vi "Update Dictionary.vi"(8 "error in (no error)":errorcluster, 9 "Variant":variant, 10 "Key":string, 11 "SMO.Dictionary in":refnum<class "SMO.Dictionary.lvclass">) -> (0 "error out":errorcluster, 3 "SMO.Dictionary out":refnum<class "SMO.Dictionary.lvclass">)   [LabVIEW 2013, in "SMO.Dictionary.lvlib" / "SMO.Dictionary.lvclass"]
uses:
  SMO.Dictionary.lvclass
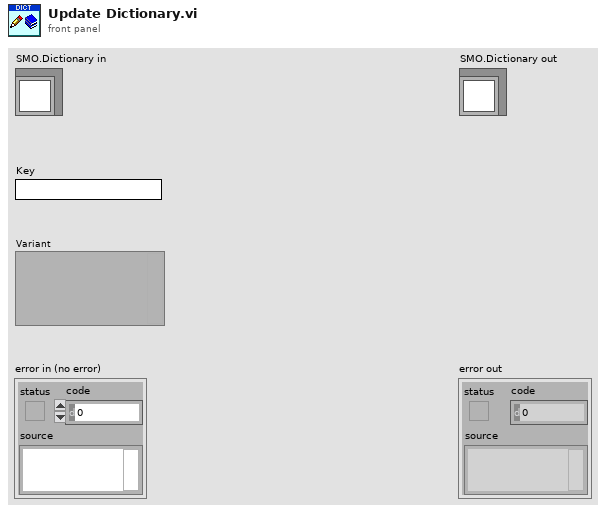
[diagram p1: front panel]
types:
  T1 = typedef "SMO.Dictionary.lvlib/SMO.Dictionary.lvclass/PublicEvents--Cluster.ctl" = cluster{"Cleared":refnum<user-event>, "Deleted":refnum<user-event>, "Updated":refnum<user-event>}
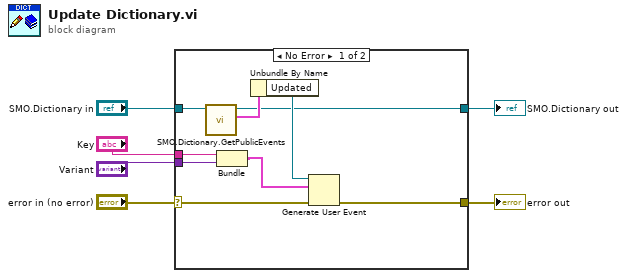
[diagram p0: block diagram]
diagram:
  n1 = case shown="No Error" "error in (no error)" {
    selector: "error in (no error)" -> [w11 w17]
    tunnel: [w10 w17] -> w5
    tunnel: [w12 w16] -> w3
    tunnel: "SMO.Dictionary in" -> [w13 w16]
    tunnel: "Key" -> [w9 _]
    tunnel: "Variant" -> [w8 _]
    frame No Error {
      n2 = call "SMO.Dictionary.GetPublicEvents.vi"("SMO.Dictionary in"=w13) -> ("Public Events"=w15:T1, "SMO.Dictionary out"=w12:refnum<class "SMO.Dictionary.lvclass">)  [unwired: 8 in, 1 out]
      n3 = Bundle("Key"=w9, "Variant"=w8) -> (w7:cluster{"Key":string, "Variant":variant})  [unwired: 1 in]
      n4 = Unbundle By Name(w15) -> ("Updated"=w14:refnum<user-event>)
      n5 = Generate User Event(user event=w14, event data cluster=w7, error in=w11) -> (error out=w10:errorcluster)  [unwired: 1 in, 1 out]
    }
    frame Error {
    }
  }
  "error out" <- w5
  "SMO.Dictionary out" <- w3
